vi "ADIS16448_RoboRIO_Teensy_FGV.vi"(0 "SerialPortRefIn":T4, 2 "IMU Angles":T2, 3 "IMU AHRS":cluster{"Pitch":dbl, "Roll":dbl, "Yaw":dbl}, 5 "error in":errorcluster, 7 "Function":T1, 8 "Operation":T3(ring), 9 "Reset":bool) -> (11 "Reset Out":bool, 13 "Function Out":T1, 14 "SerialPortRefOut":T4, 16 "IMU Angles Out":T2, 17 "IMU AHRS Out":cluster{"Pitch":dbl, "Roll":dbl, "Yaw":dbl}, 19 "error out":errorcluster)   [LabVIEW 2016, in "ADIS16448-Teensy.lvlib"]
uses:
  ADIS16448-Teensy.lvlib
  <vilib>/Rock Robotics/WPI/SerialPort/WPI_SerialPortRef.ctl
  Util_Functions.ctl
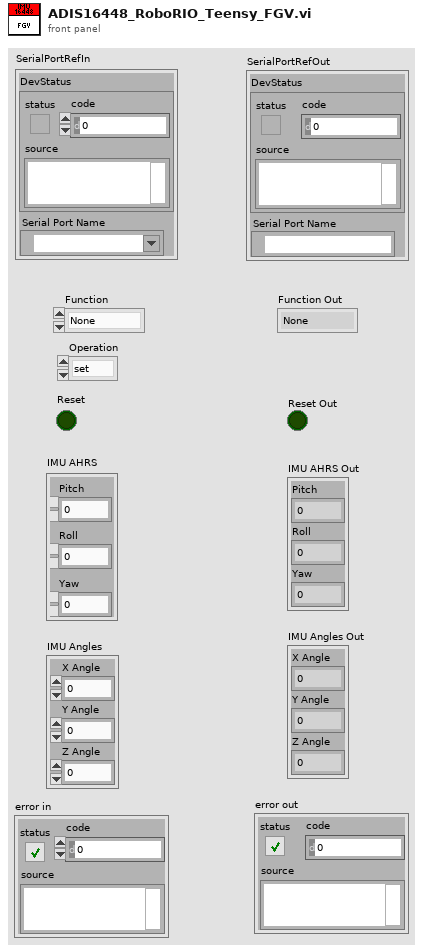
[diagram p1: front panel]
types:
  T1 = typedef "Util_Functions.ctl" = enum16{"None", "Calibrate"}
  T2 = cluster{"X Angle":dbl, "Y Angle":dbl, "Z Angle":dbl}
  T3 = enum16{"set", "get", "set reset", "set function"}
  T4 = typedef "WPI_SerialPortRef.ctl" = cluster{"DevStatus":errorcluster, "Serial Port Name":refnum<visa-resource-name>}
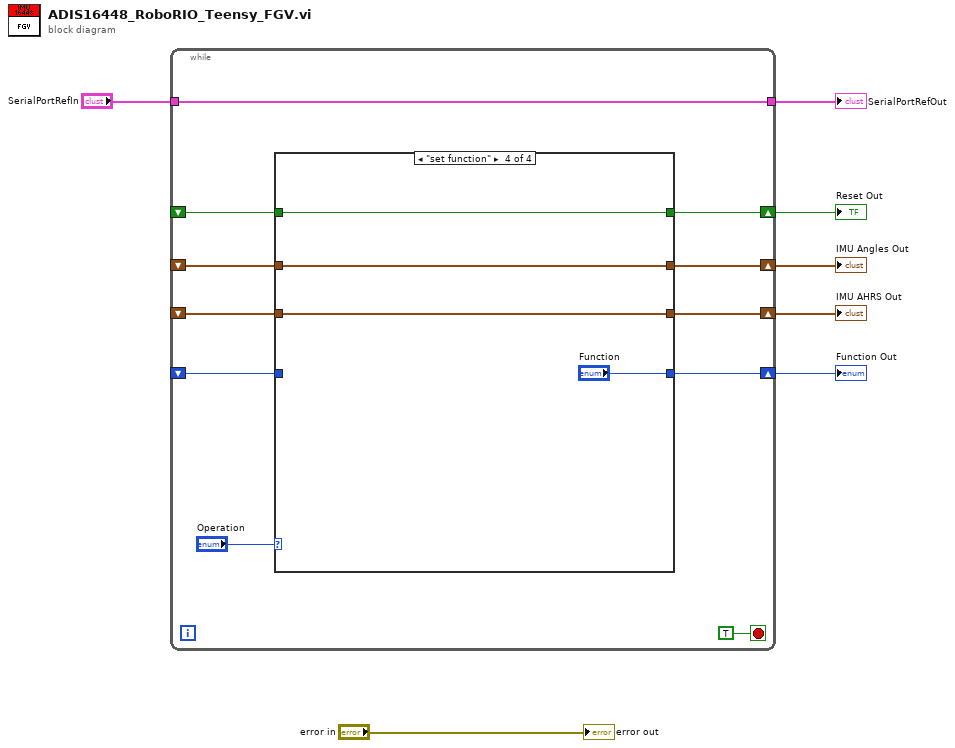
[diagram p0: block diagram]
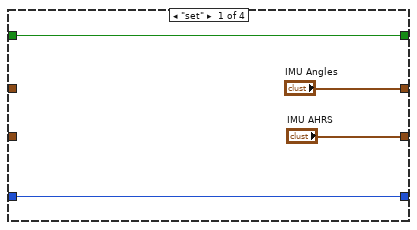
[diagram p2: hidden frame]
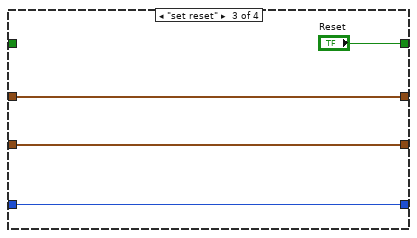
[diagram p4: hidden frame]
diagram:
  n1 = while {
    tunnel: [w17] -> w6
    tunnel: "SerialPortRefIn" -> [w17]
    shift-right: [w10] -> w3
    shift-left: _ -> [w11]
    shift-right: [w16] -> w5
    shift-left: _ -> [w15]
    shift-right: [w13] -> w4
    shift-left: _ -> [w12]
    shift-right: [w9] -> w1
    shift-left: _ -> [w8]
    stop <- TRUE stop-if-true
    n2 = case shown="\"set function\"" "Operation" {
      tunnel: ["IMU Angles" w25 w29 w33] -> w10
      tunnel: w11 -> [_ w25 w29 w33]
      tunnel: ["IMU AHRS" w26 w28 w32] -> w16
      tunnel: w15 -> [_ w26 w28 w32]
      tunnel: w12 -> [w21 w24 _ w34]
      tunnel: [w21 w24 "Reset" w34] -> w13
      tunnel: [w19 w23 w27 "Function"] -> w9
      tunnel: w8 -> [w19 w23 w27 _]
      frame "set" {
      }
      frame "get", Default {
      }
      frame "set reset" {
      }
      frame "set function" {
      }
    }
  }
  "SerialPortRefOut" <- w6
  "Reset Out" <- w4
  "IMU Angles Out" <- w3
  "IMU AHRS Out" <- w5
  "Function Out" <- w1
  "error out" <- "error in"
